vi "16TVTI-WriteHeaterOutput.vi"(2 "Heater Output (%)":dbl min=0.0 max=99.9 format="%.2f", 3 "ITC IO Info":T1={"Com Port"=1, "ISOBUS Address"=1, "GPIB Address"=1, "Communication"=enum."ISOBUS"}) -> (1 "ITC IO Info":T1={"Com Port"=1, "ISOBUS Address"=1, "GPIB Address"=1, "Communication"=enum."ISOBUS"})   [LabVIEW 2016]
doc: "Sets the heater output of the ITC."
uses:
  Equipment/Oxford Software/Oxsoft/ITCSUBS.LLB/ITCIO.ctl
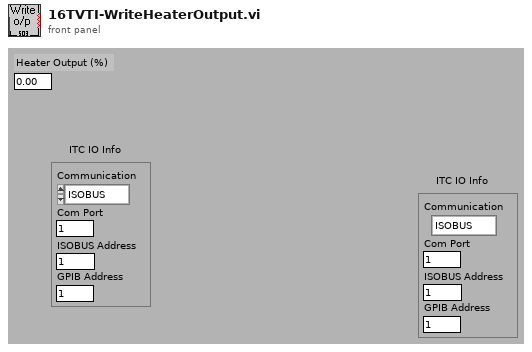
[diagram p1: front panel]
types:
  T1 = typedef "ITCIO.ctl" = cluster{"Com Port":i32, "ISOBUS Address":i32, "GPIB Address":i16, "Communication":enum16{"RS232", "ISOBUS", "GPIB", "Gateway"}}
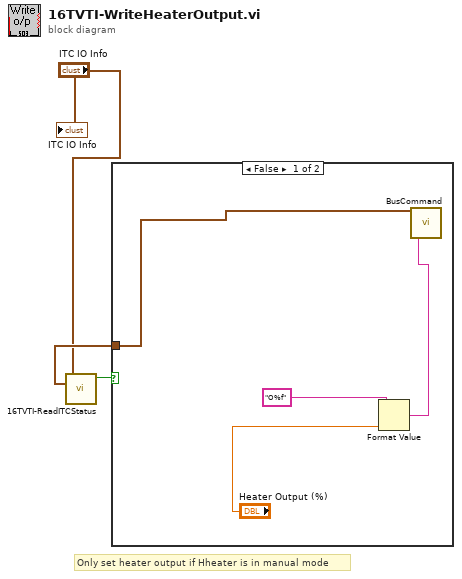
[diagram p0: block diagram]
diagram:
  # "Only set heater output if Hheater is in manual mode"
  n1 = call "16TVTI-ReadITCStatus.vi"("ITC IO Info"="ITC IO Info") -> ("Auto heat"=w3:bool, "ITC IO Info"=w2:T1)  [unwired: 4 in, 9 out]
  n2 = case shown="False" w3 {
    tunnel: w2 -> [w4 _]
    frame False {
      n3 = Format Value(format string="O%f", value (0)="Heater Output (%)") -> (output string=w7:string)  [unwired: 1 in]
      n4 = call "BusCommand.vi"("Command"=w7, "Instrument address (in)"=w4) -> ()  [unwired: 2 out]
    }
    frame True {
    }
  }
  "ITC IO Info" <- "ITC IO Info"
